vi "Dashboard Main.vi"() -> ()   [LabVIEW 2017]
uses:
  Shared/AutonomousRoutine.ctl
  <vilib>/Rock Robotics/WPI/DriverStation/WPI_DriverStationAllianceInfo.ctl
  <vilib>/Utility/miscctls.llb/LVRowAndColumnTypeDef.ctl
  <vilib>/event_ctls.llb/eventvkey.ctl
  <vilib>/Rock Robotics/WPI/Dashboard/WPI_DashboardLogging Global.vi
panel:
  in  "Camera Settings Right":T1={"Frame Rate"=30, "Compression"=30, "Size"=1, "DB Camera Config"=FALSE} {"Frame Rate" scale=1.0..30.0; "Compression" scale=100.0..-1.0; "Size" items=["640x480", "320x240", "160x120"]}
  in  "Camera Name Right":string(combo)="No Camera Selection"
  out "Camera Info":cluster{"Mbps LED":bool, "Mbps":dbl, "fps":dbl} {"fps" format="%#.1g"; "Mbps" format="%#.1g"}
  in  "Camera Settings":T1={"Frame Rate"=30, "Compression"=30, "Size"=1, "DB Camera Config"=FALSE} {"Frame Rate" scale=1.0..30.0; "Compression" scale=100.0..-1.0; "Size" items=["640x480", "320x240", "160x120"]}
  in  "TCP":refnum<k5>
  in  "Rec Mode":enum32{"Stop", "Record", "Playback"}(radio)
  out "Robot IP":string
  out "Image Message":string="Timeout in Camera Communications"
  in  "Dashboard Tab":T2(tab)
  out "NT Connection":bool
  out "Mode":T3(ring)=enum."Auto Disabled"
  out "Camera Image Right":T4(plugin-control)
  in  "DB/String 9":string
  in  "DB/String 8":string
  in  "DB/String 7":string
  in  "DB/String 6":string
  in  "DB/String 5":string
  in  "DB/String 4":string
  in  "DB/String 3":string
  in  "DB/String 2":string
  in  "DB/String 1":string
  in  "DB/String 0":string
  in  "DB/Slider 0":dbl(slide) scale=0.0..5.0
  in  "DB/Slider 1":dbl(slide) scale=0.0..5.0
  in  "DB/Slider 2":dbl(slide) scale=0.0..5.0
  in  "DB/Slider 3":dbl(slide) scale=0.0..5.0
  out "DB/LED 3":bool
  out "DB/LED 2":bool
  out "DB/LED 1":bool
  out "DB/LED 0":bool
  in  "DB/Button 3":bool
  in  "DB/Button 2":bool
  in  "DB/Button 1":bool
  in  "DB/Button 0":bool caption="New Name"
  out "Our Right Team Switch":bool
  out "Our Left Team Switch":bool
  out "Center Right Scale":bool
  out "Center Left Scale":bool
  out "Opponent Right Switch":bool
  out "Opponent Left Switch":bool
  in  "RR":T5
  in  "RL":T5
  in  "LR":T5
  in  "LL":T5
  in  "Test Slider":dbl(slide) scale=0.0..100.0 scale format="%#_3g"
  in  "On/Off":bool caption="Solenoid"
  in  "Test Name":u16(ring) items=["Select the test to run..."]
  in  "Test Tree":string(tree)
  in  "Motor":cluster{"Value":dbl, "Enable":bool} {"Value" scale=-1.0..1.0 scale format="%#_3g"}
  out "Progress":T6 {"Test Progress" scale=0.0..100.0}
  in  "Rev/Fwd":cluster{"Forward":bool, "Reverse":bool}
  in  "Test Ring":u16(ring) items=["Monochrome", "Color"]
  out "Cmd Status":string
  in  "Execute Command":bool
  in  "Command Params":string[][](table)
  in  "Command Selection":i32(listbox)
  in  "CheckList":i32(listbox)
  out "Tree":string(tree)
  out "Camera Image":T4(plugin-control)
  out "Background":bool
  in  "Camera Name":string(combo)="No Camera Selection"
  # "HW"
  # "HW"
  # "Opponent Switch"
  # "Center Scale"
  # "Our Team Switch"
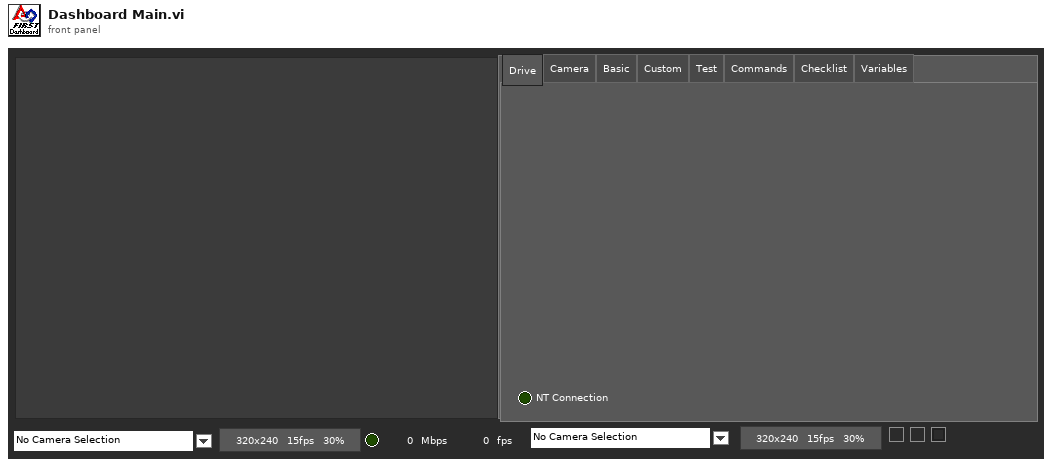
[diagram p1: front panel]
types:
  T1 = cluster{"Frame Rate":i32, "Compression":i32, "Size":u16, "DB Camera Config":bool}
  T2 = enum32{"Drive", "Camera", "Basic", "Custom", "Test", "Commands", "Checklist", "Variables"}
  T3 = enum8{"Tele-Op Disabled", "Tele-Op Enabled", "Auto Disabled", "Auto Enabled", "Test Disabled", "Test Enabled", "Disconnected", "No Code", "E-Stop"}
  T4 = typedef "IMAQ Image.ctl" = refnum<image>
  T5 = typedef "AutonomousRoutine.ctl" = enum16{"Score Scale", "Score Switch"}
  T6 = cluster{"Test Progress":u8, "Test Progress Text":string}
  T7 = cluster{"Save Path":path, "Interval (s)":dbl, "Keep":i32}
  T8 = typedef "Image Type" = u32
  T9 = cluster{"IDs":cluster{"RPC field ID":u16, "Unique ID":u16}, "String":string}
  T10 = cluster{"Error Strings":string, "Disable Counts":cluster{u16, u16}, "Rail Faults":cluster{u16, u16, u16}, "Robot IP":string, "DB Mode":u8, "Event Info":cluster{"Name":string, "Type":u8, "Number":u16, "Replay":u8}}
  T11 = cluster{"Storage":cluster{"Disk Free":u64, "RAM Block":u32, "RAM free":u32}, "CPU Utilization":cluster{"CPU % ISR":sgl, "CPU % Time Crit":sgl, "CPU % Timed Str":sgl, "CPU % High":sgl, "CPU % Above":sgl, "CPU % Normal":sgl, "CPU % Low":sgl}, "CAN":cluster{"% Bus Utilization":sgl, "Bus Off Cnt":u32, "TX_FIFO Full Cnt":u32, "Receive Error Cnt":u8, "Transmit Error Cnt":u8}, "HID":cluster{"HID Outputs":u32, "Rumble Low":u16, "Rumble High":u16}[]}
  T12 = cluster{"Status bits":cluster{"Test Mode":bool, "Autonomous":bool, "Enabled":bool, "Code Start":bool, "Brownout":bool, "Reserved 2":bool, "Reserved 3":bool, "E-Stop":bool}, "Code Trace":cluster{"Disabled":bool, "TeleOp":bool, "Auto":bool, "Test":bool}, "Controller Type":enum16{"unknown", "cRIO", "roboRio"}, "Code?":enum16{"unknown", "noCode", "code"}, "Battery V":dbl}
  T13 = cluster{"Camera Image":refnum<vi>, "Dashboard Tab":refnum<vi>, "Background":refnum<vi>, "Rec Mode":refnum<vi>, "Test Slider":refnum<vi>, "On/Off ":refnum<vi>, "Test Ring":refnum<vi>, "Rev/Fwd":refnum<vi>, "Test Name":refnum<vi>, "Motor":refnum<vi>, "Progress":refnum<vi>, "CheckList":refnum<vi>, "Tree":refnum<vi>, "Test Tree":refnum<vi>, "Command Params":refnum<vi>, "Command Selection":refnum<vi>, "Execute Command":refnum<vi>, "Cmd Status":refnum<vi>, "Camera Settings":refnum<vi>, "Camera Name":refnum<vi>, "Camera Info":refnum<vi>, "Camera Settings Right":refnum<vi>, "Camera Name Right":refnum<vi>, "Camera Image Right":refnum<vi>}
  T14 = cluster{"Camera Name":string, string, "Saved DB Images Info":cluster{"Save Path":path, "Interval (s)":dbl, "Keep":i32}}
  T15 = cluster{"Camera Name Right":string, string, "Saved DB Images Info":cluster{"Save Path":path, "Interval (s)":dbl, "Keep":i32}}
  T16 = cluster{"Operation":enum16{"Update", "Clear"}, "Color Box":u32}[]
  T17 = typedef "eventvkey.ctl" = enum16{"ASCII", "Enter", "Return", "Shift", "Ctrl", "Alt", "Cmd", "Opt", "Caps", "NumLock", "Clear", "Break", "Up", "Down", "Left", "Right", "Insert", "Delete", "Home", "End", "PageUp", "PageDown", "Escape", "Help", "Pause", "ScrollLock", "F1", "F2", "F3", "F4", "F5", "F6", "F7", "F8", "F9", "F10", "F11", "F12", "F13", "F14", "F15", "F16", "F17", "F18", "F19", "F20", "F21", "F22", "F23", "F24", "Play", "VolumeUp", "VolumeDown", "Mute", "Two Byte Char"}
  T18 = cluster{"Image Size":bool, "Image Type":bool, "Pixel Value":bool, "ROI Information":bool, "Zoom Factor":bool}
  T19 = cluster{"Operation":enum16{"Update", "Clear"}, "Color Box":u32}
  T20 = typedef "LVRowAndColumnTypeDef.ctl" = cluster{"Row":i32, "Column":i32}
  T21 = cluster{"Shift":bool, "Ctrl":bool, "Alt":bool, "Cmd":bool, "Opt":bool}
  T22 = typedef "WPI_DriverStationAllianceInfo.ctl" = enum16{"Red", "Blue", "Invalid"}
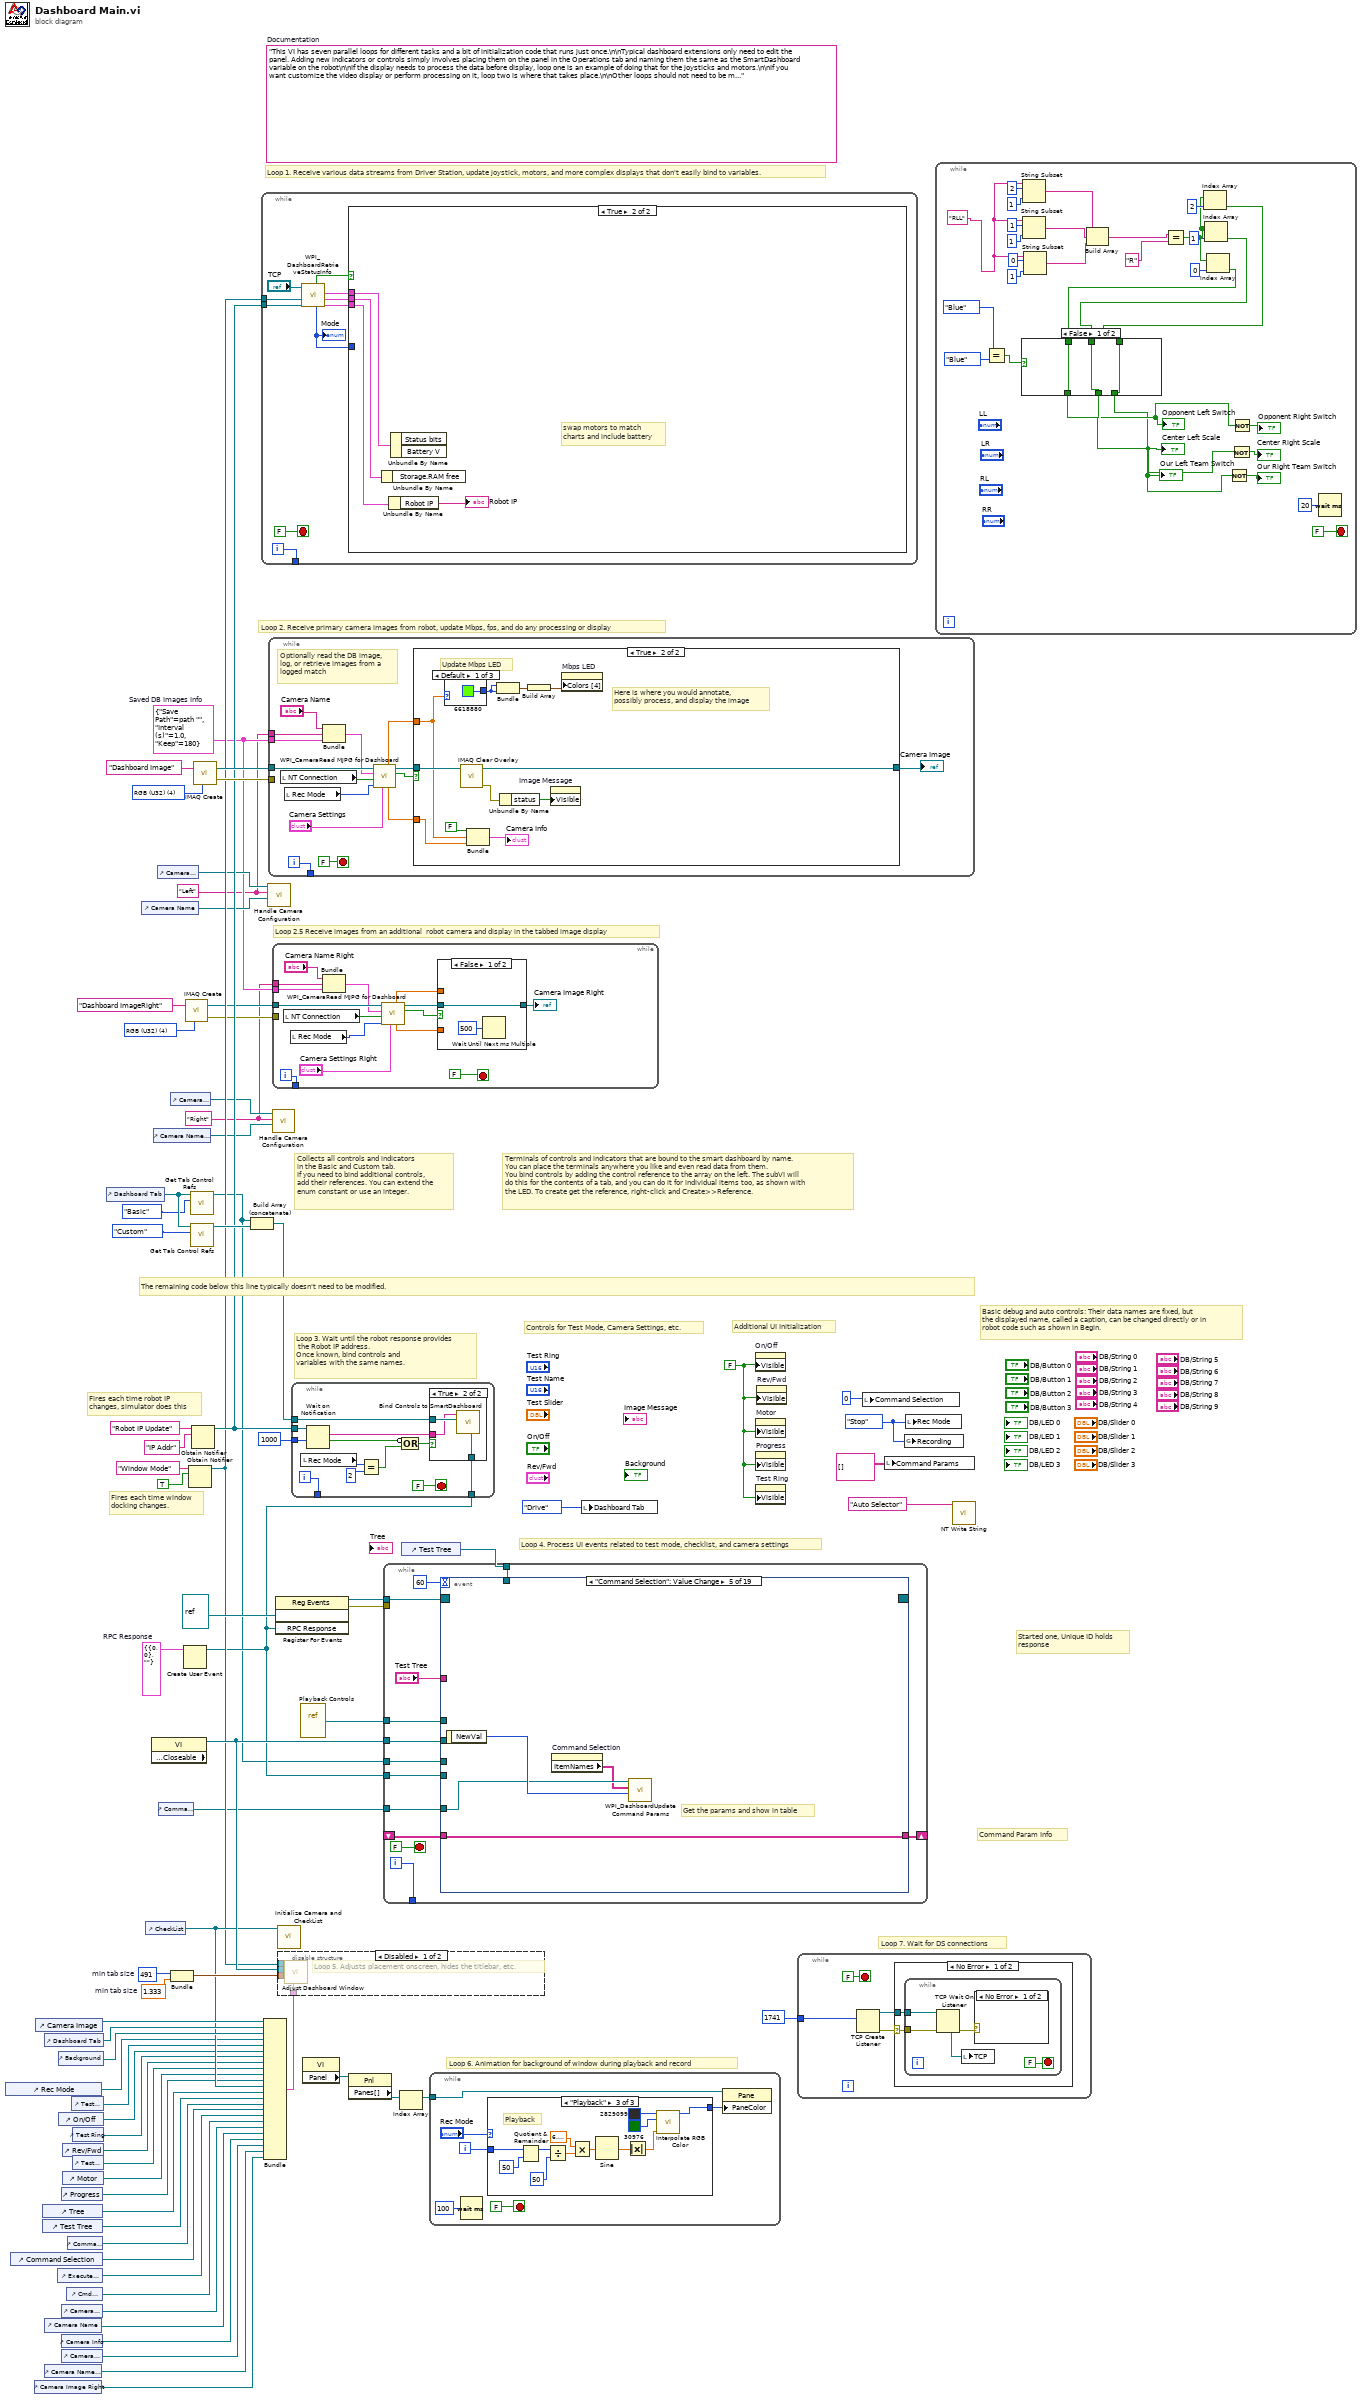
[diagram p0: block diagram]
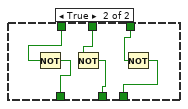
[diagram p2: hidden frame]
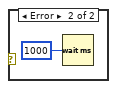
[diagram p5: hidden frame]
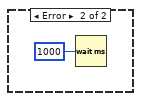
[diagram p6: hidden frame]
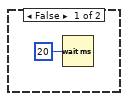
[diagram p7: hidden frame]
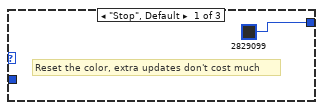
[diagram p8: hidden frame]
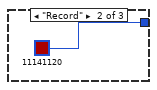
[diagram p9: hidden frame]
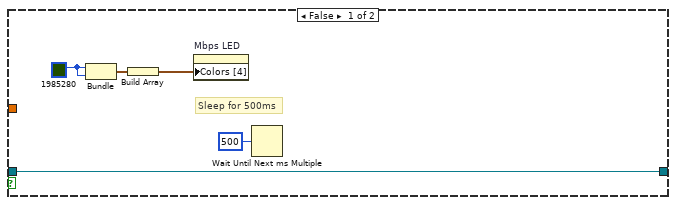
[diagram p11: hidden frame]
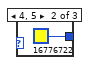
[diagram p12: hidden frame]
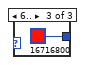
[diagram p13: hidden frame]
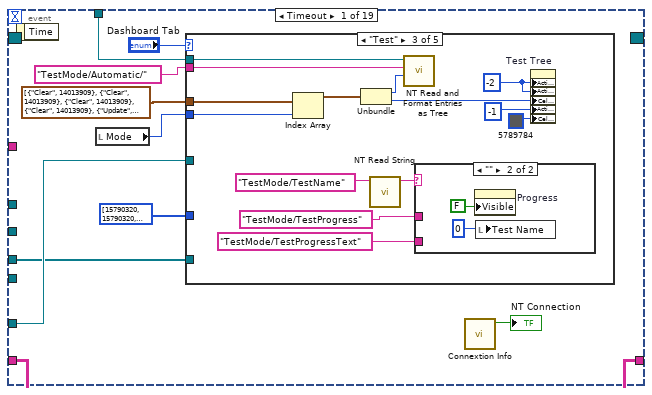
[diagram p14: hidden frame]
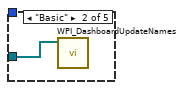
[diagram p16: hidden frame]
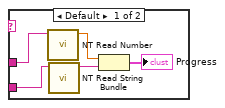
[diagram p17: hidden frame]
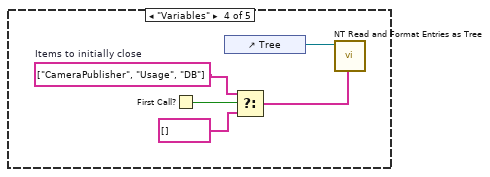
[diagram p18: hidden frame]
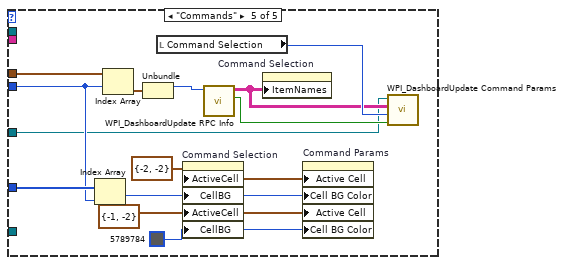
[diagram p19: hidden frame]
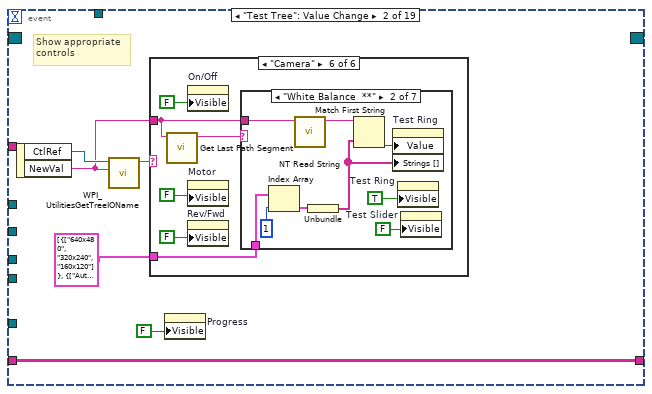
[diagram p20: hidden frame]
diagram:
  w3 = T7 {"Save Path"=path "", "Interval (s)"=1.0, "Keep"=180}  # Saved DB Images Info
  w2 = "Right"
  w1 = "Left"
  w13 = T8 4 items=["Grayscale (U8)", "Grayscale (I16)", "Grayscale (SGL)", "Complex (CSG)", "RGB (U32)", "HSL (U32)", "RGB (U64)"] ("Image Type")
  w28 = T9 {"IDs"={"RPC field ID"=0, "Unique ID"=0}, "String"=""}  # RPC Response
  w51 = 491  # min tab size
  w50 = 1.333  # min tab size
  w58 = enum32{"Stop", "Record", "Playback"}."Stop" ("Rec Mode")
  w35 = FALSE ("Visible")
  (unwired) "This VI has seven parallel loops for different tasks and a bit of initialization code that runs just once.\n\nTypical dashboard extensions only need to edit the panel. Adding new indicators or controls simply involves placing them on the panel in the Operations tab and naming them the same as the SmartDashboard variable on the robot\n\nIf the display needs to process the data before display, loop one is an example of doing that for the joysticks and motors.\n\nIf you want customize the video display or perform processing on it, loop two is where that takes place.\n\nOther loops should not need to be modified. They are pretty standard, and document the task they perform."  # Documentation
  w75 = T8 4 items=["Grayscale (U8)", "Grayscale (I16)", "Grayscale (SGL)", "Complex (CSG)", "RGB (U32)", "HSL (U32)", "RGB (U64)"] ("Image Type")
  # "Loop 2.5 Receive images from an additional  robot camera and display in the tabbed image display"
  # "Command Param Info"
  # "Started one, Unique ID holds\nresponse"
  # "Loop 7. Wait for DS connections"
  # "Basic debug and auto controls: Their data names are fixed, but\nthe displayed name, called a caption, can be changed directly or in\nrobot code such as shown in Begin."
  # "Controls for Test Mode, Camera Settings, etc."
  # "Additional UI Initialization"
  # "Loop 6. Animation for background of window during playback and record"
  # "Fires each time robot IP\nchanges, simulator does this"
  # "Fires each time window\ndocking changes."
  # "Collects all controls and indicators\nin the Basic and Custom tab.\nIf you need to bind additional controls,\nadd their references. You can extend the\nenum constant or use an integer."
  # "The remaining code below this line typically doesn't need to be modified."
  # "Loop 4. Process UI events related to test mode, checklist, and camera settings"
  # "Terminals of controls and indicators that are bound to the smart dashboard by name.\nYou can place the terminals anywhere you like and even read data from them.\nYou bind controls by adding the control reference to the array on the left. The subVI will\ndo this for the contents of a tab, and you can do it for individual items too, as shown with\nthe LED. To create get the reference, right-click and Create>>Reference."
  # "Loop 3. Wait until the robot response provides\n the Robot IP address.\nOnce known, bind controls and\nvariables with the same names."
  # "Loop 1. Receive various data streams from Driver Station, update joystick, motors, and more complex displays that don't easily bind to variables."
  # "Loop 2. Receive primary camera images from robot, update Mbps, fps, and do any processing or display"
  n1 = control-ref of="Rec Mode"() -> (w41:refnum<vi>)
  n2 = control-ref of="Command Selection"() -> (w27:refnum<vi>)
  n3 = control-ref of="Camera Image Right"() -> (w6:refnum<vi>)
  n4 = control-ref of="Camera Image"() -> (w53:refnum<vi>)
  n5 = control-ref of="Tree"() -> (w45:refnum<vi>)
  n6 = control-ref of="Test Tree"() -> (w44:refnum<vi>)
  n7 = control-ref of="Dashboard Tab"() -> (w52:refnum<vi>)
  n8 = control-ref of="Camera Name"() -> (w18:refnum<vi>)
  n9 = control-ref of="Camera Name Right"() -> (w7:refnum<vi>)
  n10 = control-ref of="Execute Command"() -> (w29:refnum<vi>)
  n11 = control-ref of="Background"() -> (w48:refnum<vi>)
  n12 = control-ref of="On/Off"() -> (w39:refnum<vi>)
  n13 = control-ref of="Progress"() -> (w36:refnum<vi>)
  n14 = control-ref of="Camera Settings"() -> (w19:refnum<vi>)
  n15 = control-ref of="Camera Info"() -> (w17:refnum<vi>)
  n16 = control-ref of="Camera Settings Right"() -> (w8:refnum<vi>)
  n17 = control-ref of="Rev/Fwd"() -> (w37:refnum<vi>)
  n18 = control-ref of="Motor"() -> (w42:refnum<vi>)
  n19 = control-ref of="Cmd Status"() -> (w23:refnum<vi>)
  n20 = control-ref of="Command Params"() -> (w30:refnum<vi>)
  n21 = control-ref of="Test Slider"() -> (w40:refnum<vi>)
  n22 = control-ref of="Test Ring"() -> (w38:refnum<vi>)
  n23 = control-ref of="Test Name"() -> (w43:refnum<vi>)
  n24 = control-ref of="Dashboard Tab"() -> (w56:refnum<vi>)
  n25 = control-ref of="Camera Name"() -> (w20:refnum<vi>)
  n26 = control-ref of="CheckList"() -> (w46:refnum<vi>)
  n27 = property class="VI" props=["Front Panel.Closeable"]() -> (reference out=w57:refnum<vi>)  [unwired: 2 in, 2 out]
  n28 = control-ref of="Camera Name Right"() -> (w9:refnum<vi>)
  n29 = control-ref of="Camera Settings"() -> (w21:refnum<vi>)
  n30 = control-ref of="Command Params"() -> (w22:refnum<vi>)
  n31 = control-ref of="Camera Settings Right"() -> (w10:refnum<vi>)
  n32 = Bundle("min tab size"=w51, "min tab size"=w50) -> (w49:cluster{"min tab size":i32, "min tab size":dbl})  [unwired: 1 in]
  n33 = Create User Event(user event datatype=w28) -> (user event=w24:refnum<user-event>)  [unwired: 1 in, 1 out]
  n34 = call "IMAQ Create"("Image Name"="Dashboard ImageRight", "Image Type"=w13) -> ("New Image"=w12:T4, "error out"=w11:errorcluster)  [unwired: 2 in, 1 out]
  n35 = Obtain Notifier(name (unnamed)="Window Mode", notification data type=TRUE) -> (notifier out=w33:refnum<notifier>)  [unwired: 2 in, 2 out]
  n36 = call <vilib>:"Get Tab Control Refs.vi"("Page Index"=T2."Basic" ("Dashboard Tab"), "TabControl in"=w56) -> ("ControlsOnPage"=w16:refnum<vi>[])  [unwired: 9 in]
  n37 = call <vilib>:"Get Tab Control Refs.vi"("Page Index"=T2."Custom" ("Dashboard Tab"), "TabControl in"=w56) -> ("ControlsOnPage"=w55:refnum<vi>[])  [unwired: 9 in]
  n38 = Obtain Notifier(name (unnamed)="Robot IP Update", notification data type="IP Addr" ("name (unnamed)")) -> (notifier out=w34:refnum<notifier>)  [unwired: 2 in, 2 out]
  n39 = call "IMAQ Create"("Image Name"="Dashboard Image", "Image Type"=w75) -> ("New Image"=w73:T4, "error out"=w72:errorcluster)  [unwired: 2 in, 1 out]
  n40 = Build Array (concatenate)(w16, w55) -> (w54:refnum<vi>[])
  n41 = while {
    tunnel: [w84] -> _
    tunnel: w34 -> [w79]
    tunnel: w33 -> [w76]
    i -> [w84]
    stop <- FALSE stop-if-true
    n42 = call <vilib>:"WPI_DashboardRetrieveStatusInfo.vi"("Binding Refnum"=w79, "Window Mode Notifier"=w76, "TCP Cnx"="TCP") -> ("Power and Errors"=w80:T10, "Robot Metrics"=w82:T11, "Status Info"=w83:T12, "Robot Mode"=w78:T3, "Process?"=w81:bool)  [unwired: 3 in, 1 out]
    "Mode" <- w78
    n43 = case shown="True" w81 {
      tunnel: w83 -> [_ w90]
      tunnel: w82 -> [_ w89]
      tunnel: w80 -> [_ w88]
      tunnel: w78 -> [_ _]
      frame False {
        n44 = Wait (ms)(milliseconds to wait=u32 20) -> ()  [unwired: 1 out]
      }
      frame True {
        # "swap motors to match\ncharts and include battery"
        n45 = Unbundle By Name(w89) -> ()  [unwired: 1 out]
        n46 = Unbundle By Name(w88) -> ("Robot IP"=→"Robot IP":string)
        n47 = Unbundle By Name(w90) -> ()  [unwired: 2 out]
      }
    }
  }
  n48 = Bundle("Camera Image"=w53, "Dashboard Tab"=w52, "Background"=w48, "Rec Mode"=w41, "Test Slider"=w40, "On/Off"=w39, "Test Ring"=w38, "Rev/Fwd"=w37, "Test Name"=w43, "Motor"=w42, "Progress"=w36, "CheckList"=w46, "Tree"=w45, "Test Tree"=w44, "Command Params"=w30, "Command Selection"=w27, "Execute Command"=w29, "Cmd Status"=w23, "Camera Settings"=w19, "Camera Name"=w18, "Camera Info"=w17, "Camera Settings Right"=w8, "Camera Name Right"=w7, "Camera Image Right"=w6) -> (w47:T13)  [unwired: 1 in]
  n49 = call "Handle Camera Configuration.vi"("CameraNameRef"=w20, "Display Name"=w1, "ClusterRef"=w21) -> ()  [unwired: 9 in]
  n50 = while {
    tunnel: w73 -> [w103]
    tunnel: w72 -> [_]
    tunnel: [w104] -> _
    tunnel: w3 -> [w94]
    tunnel: w1 -> [w91]
    i -> [w104]
    stop <- FALSE stop-if-true
    # "Optionally read the DB image,\nlog, or retrieve images from a\nlogged match"
    n51 = local read "NT Connection"() -> (w95:bool)
    n52 = local read "Rec Mode"() -> (w99:enum32{"Stop", "Record", "Playback"})
    n53 = Bundle("Camera Name"="Camera Name", w91, "Saved DB Images Info"=w94) -> (w93:T14)  [unwired: 1 in]
    n54 = call <vilib>:"WPI_CameraRead MJPG for Dashboard.vi"("Camera Settings"="Camera Settings", "Rec Mode"=w99, "NT Connection"=w95, "Capture Info"=w93, "Refnum in"=w103) -> ("Active"=w101:bool, "Refnum out"=w102:T4, "FPS"=w100:dbl, "Bandwidth (Mbps)"=w98:dbl)  [unwired: 3 in]
    n55 = case shown="True" w101 {
      tunnel: w102 -> [w106 w117]
      tunnel: w98 -> [_ w114]
      tunnel: w100 -> [_ w115]
      tunnel: [w106 w111] -> w96
      frame False {
        w108 = u32 1985280 ("Color Box")
        # "Sleep for 500ms"
        n56 = Bundle("Color Box"=w108, "Color Box"=w108) -> (w109:cluster{"Color Box":u32, "Color Box":u32})  [unwired: 1 out]
        n57 = Build Array(w109) -> (w107:cluster{"Color Box":u32, "Color Box":u32}[])
        n58 = property on="Mbps LED" class="Bool (strict)"("Colors [4]"=w107) -> ()  [unwired: 2 in, 2 out]
        n59 = Wait Until Next ms Multiple(millisecond multiple=u32 500) -> ()  [unwired: 1 out]
      }
      frame True {
        # "Here is where you would annotate,\npossibly process, and display the image"
        # "Update Mbps LED"
        n60 = case shown="Default" w114 {
          tunnel: [u32 6618880 ("Color Box") u32 16776722 ("Color Box") u32 16716800 ("Color Box")] -> w118
          frame Default {
          }
          frame 4, 5 {
          }
          frame 6.. {
          }
        }
        n61 = call "IMAQ Clear Overlay"("Image"=w117) -> ("error out"=w120:errorcluster, "Image Out"=w111:T4)  [unwired: 2 in, 7 out]
        n62 = Bundle(FALSE, "Bandwidth (Mbps)"=w114, "FPS"=w115) -> (→"Camera Info":cluster{bool, "Bandwidth (Mbps)":dbl, "FPS":dbl})  [unwired: 1 in]
        n63 = Bundle("Color Box"=w118, "Color Box"=w118) -> (w119:cluster{"Color Box":u32, "Color Box":u32})  [unwired: 1 out]
        n64 = Unbundle By Name(w120) -> ("status"=w121:bool)
        n65 = Build Array(w119) -> (w116:cluster{"Color Box":u32, "Color Box":u32}[])
        n66 = property on="Image Message" class="Str"("Visible"=w121) -> ()  [unwired: 2 in, 2 out]
        n67 = property on="Mbps LED" class="Bool (strict)"("Colors [4]"=w116) -> ()  [unwired: 2 in, 2 out]
      }
    }
    "Camera Image" <- w96
  }
  n68 = call "Handle Camera Configuration.vi"("CameraNameRef"=w9, "Display Name"=w2, "ClusterRef"=w10) -> ()  [unwired: 9 in]
  n69 = while {
    tunnel: w12 -> [w139]
    tunnel: w11 -> [_]
    tunnel: [w134] -> _
    tunnel: w3 -> [w128]
    tunnel: w2 -> [w125]
    i -> [w134]
    stop <- FALSE stop-if-true
    n70 = local read "NT Connection"() -> (w129:bool)
    n71 = local read "Rec Mode"() -> (w138:enum32{"Stop", "Record", "Playback"})
    n72 = Bundle("Camera Name Right"="Camera Name Right", w125, "Saved DB Images Info"=w128) -> (w127:T15)  [unwired: 1 in]
    n73 = call <vilib>:"WPI_CameraRead MJPG for Dashboard.vi"("Camera Settings"="Camera Settings Right", "Rec Mode"=w138, "NT Connection"=w129, "Capture Info"=w127, "Refnum in"=w139) -> ("Active"=w133:bool, "Refnum out"=w136:T4, "FPS"=w131:dbl, "Bandwidth (Mbps)"=w132:dbl)  [unwired: 3 in]
    n74 = case shown="False" w133 {
      tunnel: w136 -> [w140 w142]
      tunnel: w132 -> [_ _]
      tunnel: w131 -> [_ _]
      tunnel: [w140 w142] -> w130
      frame False {
        n75 = Wait Until Next ms Multiple(millisecond multiple=u32 500) -> ()  [unwired: 1 out]
      }
      frame True {
      }
    }
    "Camera Image Right" <- w130
  }
  n76 = register-events(refnum<vi> refnum, w24) -> (reference out=w62:refnum<event-registration>, error out=w61:errorcluster)  [unwired: 2 in]
  n77 = call "Initialize Camera and CheckList.vi"("ListBox in"=w46) -> ()  [unwired: 11 in]
  n78 = disable-structure shown="Disabled" {
    disable-tunnel: w57 -> [w146 _]
    disable-tunnel: w49 -> [w145 _]
    disable-tunnel: w47 -> [w144 _]
    disable-tunnel: w33 -> [w143 _]
    frame Disabled {
      # "Loop 5. Adjusts placement onscreen, hides the titlebar, etc."
      n79 = call "Adjust Dashboard Window.vi"("Sizing Refnums"=w144, "Size Constraints"=w145, "VI"=w146, "WIn Mode"=w143) -> ()  [unwired: 8 in]
    }
    frame Enabled {
    }
  }
  n80 = while {
    tunnel: w54 -> [w158]
    tunnel: w34 -> [w156]
    tunnel: [w154] -> _
    tunnel: u32 1000 ("milliseconds to wait") -> [w153]
    tunnel: w24 -> [w147]
    i -> [w154]
    stop <- FALSE stop-if-true
    n81 = local read "Rec Mode"() -> (w149:enum32{"Stop", "Record", "Playback"})
    n82 = Wait on Notification(notifier=w156, timeout in ms (-1)=w153) -> (notification=w155:string, timed out?=w151:bool)  [unwired: 2 in, 2 out]
    n83 = Equal?(x=w149, y=u16 2 ("Rec Mode")) -> (x = y?=w150:bool)
    n84 = Compound Arithmetic op=OR(invert w151, w150) -> (w152:bool)
    n85 = case shown="True" w152 {
      tunnel: w158 -> [_ w161]
      tunnel: w155 -> [_ w160]
      tunnel: w147 -> [_ w159]
      frame False {
      }
      frame True {
        n86 = call <vilib>:"Bind Controls to SmartDashboard.vi"("RPC ref"=w159, "Bound Control Refs"=w161, "Server IP Address"=w160) -> ()  [unwired: 9 in]
      }
    }
  }
  n87 = vi-ref "Playback Controls.vi"() -> (w63:refnum<vi>)
  n88 = property class="VI"() -> ("Panel"=w65:refnum<vi>)  [unwired: 2 in, 2 out]
  n89 = property class="Pnl"(reference=w65) -> ("Panes[]"=w66:refnum<vi>[])  [unwired: 1 in, 2 out]
  n90 = Index Array(array=w66) -> (element=w64:refnum<vi>)  [unwired: 1 in]
  n91 = control-ref of="Test Tree"() -> (w67:refnum<vi>)
  n92 = while {
    tunnel: [w171] -> _
    tunnel: w67 -> [w170]
    tunnel: w63 -> [w169]
    tunnel: w62 -> [w168]
    tunnel: w61 -> [_]
    tunnel: w57 -> [w167]
    tunnel: w24 -> [w166]
    tunnel: w22 -> [w165]
    shift-right: [w164] -> _
    shift-left: _ -> [w163]
    tunnel: w16 -> [w162]
    i -> [w171]
    stop <- FALSE stop-if-true
    n93 = event shown="[4] \"Command Selection\": Value Change" {
      selector: w168 -> [_ _ _ _ _ _ _ _ _ _ _ _ _ _ _ _ _ _ _]
      dyn-events: [_ _ _ _ _ _ _ _ _ _ _ _ _ _ w425 _ _ _ _] -> _
      timeout: u32 60 ("milliseconds to wait") -> [_ _ _ _ _ _ _ _ _ _ _ _ _ _ _ _ _ _ _]
      tunnel: w170 -> [w183 _ _ _ _ _ _ _ _ _ _ _ _ _ _ _ _ _ _]
      tunnel: "Test Tree" -> [_ _ _ _ _ _ _ _ _ w392 w400 w402 w406 w414 _ _ _ _ _]
      tunnel: w169 -> [_ _ _ _ _ _ _ _ _ _ _ _ _ _ w427 _ w445 _ _]
      tunnel: w167 -> [_ _ _ _ _ _ _ _ _ _ _ _ _ _ w423 _ _ _ _]
      tunnel: w166 -> [_ _ _ _ _ _ _ _ _ _ _ _ _ _ w421 _ _ _ _]
      tunnel: w165 -> [w178 _ _ _ w343 _ _ _ _ _ _ _ _ _ _ _ _ _ _]
      tunnel: [w177 w226 w328 w333 w341 w350 w360 w367 w379 w391 w398 w401 w405 w413 w420 w440 w442 w446 w459] -> w164
      tunnel: w163 -> [w177 w226 w328 w333 w341 _ _ w367 w379 w391 w398 w401 w405 w413 w420 w440 w442 w446 w459]
      tunnel: w162 -> [w175 _ _ _ _ _ _ _ _ _ _ _ _ _ _ _ _ _ _]
      event Timeout {
        n94 = event-data() -> ()  [unwired: 1 in, 1 out]
        n95 = local read "Mode"() -> (w180:T3)
        n96 = case shown="\"Test\"" "Dashboard Tab" {
          tunnel: w183 -> [_ _ w199 _ _]
          tunnel: "TestMode/Automatic/" ("Name Pattern") -> [_ _ w198 _ _]
          tunnel: T16 [{"Operation"=enum."Clear", "Color Box"=14013909}, {"Operation"=enum."Clear", "Color Box"=14013909}, {"Operation"=enum."Clear", "Color Box"=14013909}, {"Operation"=enum."Clear", "Color Box"=14013909}, {"Operation"=enum."Update", "Color Box"=14013909}, {"Operation"=enum."Update", "Color Box"=16777215}, {"Operation"=enum."Clear", "Color Box"=14013909}, {"Operation"=enum."Clear", "Color Box"=14013909}, {"Operation"=enum."Clear", "Color Box"=14013909}] -> [_ _ w191 _ w219]
          tunnel: w180 -> [_ _ w190 _ w218]
          tunnel: u32[] [15790320, 15790320, 15790320, 15790320, 16777215, 16777215, 15790320, 15790320, 15790320] -> [_ _ _ _ w224]
          tunnel: w178 -> [_ _ _ _ w212]
          tunnel: w175 -> [_ w185 _ _ _]
          frame "Custom", Default {
          }
          frame "Basic" {
            n97 = call <vilib>:"WPI_DashboardUpdateNames.vi"("Controls on Tab"=w185) -> ()  [unwired: 11 in]
          }
          frame "Test" {
            w197 = -2 ("Active Item:Row Number")
            n98 = Index Array(array=w191, index=w190) -> (element=w192:T19)
            n99 = Unbundle(w192) -> ("Operation"=w193:enum16{"Update", "Clear"}, "Color Box"=w194:u32)
            n100 = call <vilib>:"NT Read String.vi"("Name"="TestMode/TestName") -> ("String"=w188:string)  [unwired: 9 in, 1 out]
            n101 = call <vilib>:"NT Read and Format Entries as Tree.vi"("Operation"=w193, "Name Pattern"=w198, "Tree Refnum"=w199) -> ()  [unwired: 7 in, 2 out]
            n102 = case shown="\"\"" w188 {
              tunnel: "TestMode/TestProgress" ("Name") -> [w201 _]
              tunnel: "TestMode/TestProgressText" ("Name") -> [w200 _]
              frame Default {
                n103 = call <vilib>:"NT Read Number.vi"("Name"=w201) -> ("Numeric"=w202:dbl)  [unwired: 9 in, 1 out]
                n104 = call <vilib>:"NT Read String.vi"("Name"=w200) -> ("String"=w203:string)  [unwired: 9 in, 1 out]
                n105 = Bundle("Numeric"=w202, "String"=w203) -> (→"Progress":cluster{"Numeric":dbl, "String":string})  [unwired: 1 in]
              }
              frame "" {
                n106 = property on="Progress" class="Clust (strict)"("Visible"=FALSE) -> ()  [unwired: 2 in, 2 out]
                n107 = local write "Test Name"(u16 0) -> ()
              }
            }
            n108 = property on="Test Tree" class="Tree (strict)"("Active Item Row Number"=w197, "ActiveColNum"=w197, "CellBG"=w194, "Active Item Row Number"=-1 ("Active Item:Row Number"), "CellBG"=u32 5789784 ("Color Box")) -> ()  [unwired: 2 in, 2 out]
          }
          frame "Variables" {
            w209 = string[] ["CameraPublisher", "Usage", "DB"]  # Items to initially close
            n109 = First Call?() -> (First Call?: T/F=w210:bool)
            n110 = control-ref of="Tree"() -> (w211:refnum<vi>)
            n111 = Select(t=w209, s=w210, f=string[] []) -> (s? t:f=w207:string[])
            n112 = call <vilib>:"NT Read and Format Entries as Tree.vi"("Tags to  Close"=w207, "Tree Refnum"=w211) -> ()  [unwired: 8 in, 2 out]
          }
          frame "Commands" {
            w220 = u32 5789784 ("Color Box")
            w221 = T20 {"Row"=-1, "Column"=-2} ("Active Cell:Active Cell")
            w223 = T20 {"Row"=-2, "Column"=-2} ("Active Cell:Active Cell")
            n113 = Index Array(array=w224, index=w218) -> (element=w222:u32)
            n114 = Index Array(array=w219, index=w218) -> (element=w217:T19)
            n115 = Unbundle(w217) -> ("Operation"=w216:enum16{"Update", "Clear"})  [unwired: 1 out]
            n116 = local read "Command Selection"() -> (w215:i32)
            n117 = property on="Command Selection" class="MCListbox (strict)"("ActiveCell"=w223, "CellBG"=w222, "ActiveCell"=w221, "CellBG"=w220) -> ()  [unwired: 2 in, 2 out]
            n118 = call <vilib>:"WPI_DashboardUpdate RPC Info.vi"("Operation"=w216) -> ("update"=w214:bool, "commands"=w213:string[][])  [unwired: 9 in]
            n119 = property on="Command Selection" class="MCListbox (strict)"("ItemNames"=w213) -> ()  [unwired: 2 in, 2 out]
            n120 = property on="Command Params" class="Tbl (strict)"("Active Cell"=w223, "Cell BG Color"=w222, "Active Cell"=w221, "Cell BG Color"=w220) -> ()  [unwired: 2 in, 2 out]
            n121 = call <vilib>:"WPI_DashboardUpdate Command Params.vi"("Update"=w214, "NewVal"=w215, "Commands"=w213, "Param Tbl"=w212) -> ()  [unwired: 7 in, 1 out]
          }
        }
        n122 = call <vilib>:"Connextion Info.vi"() -> ("Connected"=→"NT Connection":bool)  [unwired: 10 in, 1 out]
      }
      event "Test Tree": Value Change {
        # "Show appropriate\ncontrols"
        n123 = event-data() -> ("CtlRef"=w229:refnum<vi>, "NewVal"=w227:string)  [unwired: 1 in]
        n124 = call <vilib>:"WPI_UtilitiesGetTreeIOName.vi"("NewVal"=w227, "TreeControl in"=w229) -> ("I/O Name"=w230:string)  [unwired: 9 in]
        n125 = case shown="\"Camera\"" w230 {
          selector: w230 -> [_ w237 _ w259 w268 _]
          tunnel: w227 -> [_ _ w256 w258 _ w275]
          tunnel: cluster{string[]}[] [{["640x480", "320x240", "160x120"]}, {["Auto", "Fixed indoor", "Fixed outdoor 1", "Fixed outdoor 2", "Fixed fluorescent 1", "Fixed fluorescent 2", "Hold current"]}, {["Auto", "Flicker-free 50 Hz", "Flicker-free 60 Hz", "Hold current"]}, {["None", "Prioritize frame rate", "Prioritize image quality"]}, {["Monochrome", "Color"]}] -> [_ _ _ _ _ w274]
          frame Default {
            w232 = FALSE ("Visible")
            w231 = FALSE ("Visible")
            n126 = property on="Motor" class="Clust (strict)"("Visible"=w231) -> ()  [unwired: 2 in, 2 out]
            n127 = property on="Test Ring" class="Ring (strict)"("Visible"=w231) -> ()  [unwired: 2 in, 2 out]
            n128 = property on="Rev/Fwd" class="Clust (strict)"("Visible"=w232) -> ()  [unwired: 2 in, 2 out]
            n129 = property on="On/Off" class="Bool (strict)"("Visible"=w232) -> ()  [unwired: 2 in, 2 out]
            n130 = property on="Test Slider" class="Slide (strict)"("Visible"=w232) -> ()  [unwired: 2 in, 2 out]
          }
          frame "Analog Out", "Motor", "PWM" {
            w238 = FALSE ("Visible")
            n131 = case shown="\"Analog Out\"" w237 {
              tunnel: [1.0 ("Value") -1.0 ("Value") 0.0 ("Value")] -> w236
              tunnel: [255.0 ("Value") 1.0 ("Value") 5.0 ("Value")] -> w235
              tunnel: [128.0 ("Value") 0.0 ("Value") 0.0 ("Value")] -> w234
              tunnel: [64.0 ("Value") 0.5 ("Value") 1.0 ("Value")] -> w233
              frame "PWM" {
              }
              frame "Motor", Default {
              }
              frame "Analog Out" {
              }
            }
            n132 = property on="Motor" class="Clust (strict)"("Visible"=TRUE) -> ()  [unwired: 2 in, 2 out]
            n133 = property on="Value" class="Slide (strict)"("Value"=w234, "Scale.Minimum"=w236, "Scale.Maximum"=w235, "Scale.Increment"=w233) -> ()  [unwired: 2 in, 2 out]
            n134 = property on="On/Off" class="Bool (strict)"("Visible"=w238) -> ()  [unwired: 2 in, 2 out]
            n135 = property on="Test Slider" class="Slide (strict)"("Visible"=w238) -> ()  [unwired: 2 in, 2 out]
            n136 = property on="Test Ring" class="Ring (strict)"("Visible"=w238) -> ()  [unwired: 2 in, 2 out]
            n137 = property on="Rev/Fwd" class="Clust (strict)"("Visible"=w238) -> ()  [unwired: 2 in, 2 out]
          }
          frame "Servo" {
            w254 = FALSE ("Visible")
            n138 = call <vilib>:"NT Read Number.vi"("Name"=w256) -> ("Numeric"=w255:dbl)  [unwired: 9 in, 1 out]
            n139 = property on="Test Slider" class="Slide (strict)"("Visible"=TRUE, "Scale.Maximum"=170.0 ("Scale.Range:Maximum")) -> ()  [unwired: 2 in, 2 out]
            n140 = local write "Test Slider"(w255) -> ()
            n141 = property on="Motor" class="Clust (strict)"("Visible"=w254) -> ()  [unwired: 2 in, 2 out]
            n142 = property on="Rev/Fwd" class="Clust (strict)"("Visible"=w254) -> ()  [unwired: 2 in, 2 out]
            n143 = property on="On/Off" class="Bool (strict)"("Visible"=w254) -> ()  [unwired: 2 in, 2 out]
            n144 = property on="Test Ring" class="Ring (strict)"("Visible"=w254) -> ()  [unwired: 2 in, 2 out]
          }
          frame "Relay", "Solenoid" {
            w257 = FALSE ("Visible")
            n145 = property on="Motor" class="Clust (strict)"("Visible"=w257) -> ()  [unwired: 2 in, 2 out]
            n146 = property on="Test Slider" class="Slide (strict)"("Visible"=w257) -> ()  [unwired: 2 in, 2 out]
            n147 = Search and Replace String(input string=w258, search string="/Value  **", replace string="/Direction") -> (result string=w264:string)  [unwired: 5 in, 3 out]
            n148 = property on="Test Ring" class="Ring (strict)"("Visible"=w257) -> ()  [unwired: 2 in, 2 out]
            n149 = call <vilib>:"NT Read String.vi"("Name"=w264) -> ("String"=w262:string)  [unwired: 9 in, 1 out]
            n150 = Equal?(x="Both directions", y=w262) -> (x = y?=w260:bool)
            n151 = Not(x=w260) -> (.not. x?=w261:bool)
            n152 = property on="Rev/Fwd" class="Clust (strict)"("Visible"=w260) -> ()  [unwired: 2 in, 2 out]
            n153 = property on="On/Off" class="Bool (strict)"("Visible"=w261, "Caption.Text"=w259) -> ()  [unwired: 2 in, 2 out]
          }
          frame "Compressor", "Digital Out" {
            w267 = FALSE ("Visible")
            # "Get direction and finish"
            n154 = property on="Motor" class="Clust (strict)"("Visible"=w267) -> ()  [unwired: 2 in, 2 out]
            n155 = property on="Test Slider" class="Slide (strict)"("Visible"=w267) -> ()  [unwired: 2 in, 2 out]
            n156 = property on="Test Ring" class="Ring (strict)"("Visible"=w267) -> ()  [unwired: 2 in, 2 out]
            n157 = property on="On/Off" class="Bool (strict)"("Visible"=TRUE, "Caption.Text"=w268) -> ()  [unwired: 2 in, 2 out]
            n158 = property on="Rev/Fwd" class="Clust (strict)"("Visible"=FALSE) -> ()  [unwired: 2 in, 2 out]
          }
          frame "Camera" {
            n159 = call <vilib>:"Get Last Path Segment.vi"("String in"=w275) -> ("String out"=w276:string)  [unwired: 10 in]
            n160 = property on="On/Off" class="Bool (strict)"("Visible"=FALSE) -> ()  [unwired: 2 in, 2 out]
            n161 = property on="Motor" class="Clust (strict)"("Visible"=FALSE) -> ()  [unwired: 2 in, 2 out]
            n162 = property on="Rev/Fwd" class="Clust (strict)"("Visible"=FALSE) -> ()  [unwired: 2 in, 2 out]
            n163 = case shown="\"White Balance  **\"" w276 {
              tunnel: w275 -> [w282 w291 w300 w309 w318 _ w324]
              tunnel: w274 -> [w280 w288 w297 w306 w315 _ _]
              frame "Size  **" {
                n164 = Index Array(array=w280) -> (element=w279:cluster{string[]})  [unwired: 1 in]
                n165 = call <vilib>:"NT Read String.vi"("Name"=w282) -> ("String"=w281:string)  [unwired: 9 in, 1 out]
                n166 = Unbundle(w279) -> (w277:string[])
                n167 = Match First String(2:w277, 3:w281) -> (0:w278:i32)  [unwired: 1 out]
                n168 = property on="Test Ring" class="Ring (strict)"("Value"=w278, "Strings []"=w277) -> ()  [unwired: 2 in, 2 out]
                n169 = property on="Test Ring" class="Ring (strict)"("Visible"=TRUE) -> ()  [unwired: 2 in, 2 out]
                n170 = property on="Test Slider" class="Slide (strict)"("Visible"=FALSE) -> ()  [unwired: 2 in, 2 out]
              }
              frame "White Balance  **" {
                n171 = Index Array(array=w288, index=1) -> (element=w289:cluster{string[]})
                n172 = call <vilib>:"NT Read String.vi"("Name"=w291) -> ("String"=w290:string)  [unwired: 9 in, 1 out]
                n173 = Unbundle(w289) -> (w286:string[])
                n174 = Match First String(2:w286, 3:w290) -> (0:w285:i32)  [unwired: 1 out]
                n175 = property on="Test Ring" class="Ring (strict)"("Value"=w285, "Strings []"=w286) -> ()  [unwired: 2 in, 2 out]
                n176 = property on="Test Ring" class="Ring (strict)"("Visible"=TRUE) -> ()  [unwired: 2 in, 2 out]
                n177 = property on="Test Slider" class="Slide (strict)"("Visible"=FALSE) -> ()  [unwired: 2 in, 2 out]
              }
              frame "Exposure  **" {
                n178 = Index Array(array=w297, index=2) -> (element=w298:cluster{string[]})
                n179 = call <vilib>:"NT Read String.vi"("Name"=w300) -> ("String"=w299:string)  [unwired: 9 in, 1 out]
                n180 = Unbundle(w298) -> (w294:string[])
                n181 = Match First String(2:w294, 3:w299) -> (0:w295:i32)  [unwired: 1 out]
                n182 = property on="Test Ring" class="Ring (strict)"("Value"=w295, "Strings []"=w294) -> ()  [unwired: 2 in, 2 out]
                n183 = property on="Test Ring" class="Ring (strict)"("Visible"=TRUE) -> ()  [unwired: 2 in, 2 out]
                n184 = property on="Test Slider" class="Slide (strict)"("Visible"=FALSE) -> ()  [unwired: 2 in, 2 out]
              }
              frame "Exposure Priority  **" {
                n185 = Index Array(array=w306, index=3) -> (element=w307:cluster{string[]})
                n186 = call <vilib>:"NT Read String.vi"("Name"=w309) -> ("String"=w308:string)  [unwired: 9 in, 1 out]
                n187 = Unbundle(w307) -> (w303:string[])
                n188 = Match First String(2:w303, 3:w308) -> (0:w304:i32)  [unwired: 1 out]
                n189 = property on="Test Ring" class="Ring (strict)"("Value"=w304, "Strings []"=w303) -> ()  [unwired: 2 in, 2 out]
                n190 = property on="Test Ring" class="Ring (strict)"("Visible"=TRUE) -> ()  [unwired: 2 in, 2 out]
                n191 = property on="Test Slider" class="Slide (strict)"("Visible"=FALSE) -> ()  [unwired: 2 in, 2 out]
              }
              frame "Color Enable  **" {
                n192 = Index Array(array=w315, index=4) -> (element=w316:cluster{string[]})
                n193 = call <vilib>:"NT Read String.vi"("Name"=w318) -> ("String"=w317:string)  [unwired: 9 in, 1 out]
                n194 = Unbundle(w316) -> (w312:string[])
                n195 = Match First String(2:w312, 3:w317) -> (0:w313:i32)  [unwired: 1 out]
                n196 = property on="Test Ring" class="Ring (strict)"("Value"=w313, "Strings []"=w312) -> ()  [unwired: 2 in, 2 out]
                n197 = property on="Test Ring" class="Ring (strict)"("Visible"=TRUE) -> ()  [unwired: 2 in, 2 out]
                n198 = property on="Test Slider" class="Slide (strict)"("Visible"=FALSE) -> ()  [unwired: 2 in, 2 out]
              }
              frame Default {
                n199 = property on="Test Ring" class="Ring (strict)"("Visible"=FALSE) -> ()  [unwired: 2 in, 2 out]
                n200 = property on="Test Slider" class="Slide (strict)"("Visible"=FALSE) -> ()  [unwired: 2 in, 2 out]
              }
              frame "Brightness  **", "Color Level  **", "Compression  **", "FPS  **", "Sharpness  **" {
                n201 = call <vilib>:"NT Read Number.vi"("Name"=w324) -> ("Numeric"=w323:dbl)  [unwired: 9 in, 1 out]
                n202 = local write "Test Slider"(w323) -> ()
                n203 = property on="Test Slider" class="Slide (strict)"("Visible"=TRUE, "Scale.Maximum"=100.0 ("Scale.Range:Maximum")) -> ()  [unwired: 2 in, 2 out]
                n204 = property on="Test Ring" class="Ring (strict)"("Visible"=FALSE) -> ()  [unwired: 2 in, 2 out]
              }
            }
          }
        }
        n205 = property on="Progress" class="Clust (strict)"("Visible"=FALSE) -> ()  [unwired: 2 in, 2 out]
      }
      event "Test Name": Mouse Enter {
        # "Populate the ring with the list of tests"
        n206 = event-data() -> ()  [unwired: 1 in, 1 out]
        n207 = call <vilib>:"NT Read String Array.vi"("Name"="TestMode/TestList") -> ("String Array"=w332:string[])  [unwired: 9 in, 1 out]
        n208 = Build Array (concatenate)("Select the test to run...", w332) -> (w331:string[])
        n209 = property on="Test Name" class="Ring (strict)"("Strings []"=w331) -> ()  [unwired: 2 in, 2 out]
      }
      event "Test Name": Value Change {
        w334 = FALSE ("Visible")
        # "Tell the robot the test name to run"
        n210 = event-data() -> ("NewVal"=w338:u16)  [unwired: 1 in]
        n211 = property on="Test Name" class="Ring (strict)"() -> ("Strings []"=w339:string[])  [unwired: 2 in, 2 out]
        n212 = local write "Progress"(T6 {"Test Progress"=0, "Test Progress Text"=""} ("Progress")) -> ()
        n213 = Index Array(array=w339, index=w338) -> (element=w337:string)
        n214 = call <vilib>:"NT Write String.vi"("String"=w337, "Name"="TestMode/TestName") -> ()  [unwired: 9 in, 1 out]
        n215 = property on="Progress" class="Clust (strict)"("Visible"=TRUE) -> ()  [unwired: 2 in, 2 out]
        n216 = property on="Motor" class="Clust (strict)"("Visible"=w334) -> ()  [unwired: 2 in, 2 out]
        n217 = property on="Test Slider" class="Slide (strict)"("Visible"=w334) -> ()  [unwired: 2 in, 2 out]
        n218 = property on="On/Off" class="Bool (strict)"("Visible"=w334) -> ()  [unwired: 2 in, 2 out]
        n219 = property on="Rev/Fwd" class="Clust (strict)"("Visible"=w334) -> ()  [unwired: 2 in, 2 out]
        n220 = property on="Test Ring" class="Ring (strict)"("Visible"=w334) -> ()  [unwired: 2 in, 2 out]
      }
      event "Command Selection": Value Change {
        # "Get the params and show in table"
        n221 = event-data() -> ("NewVal"=w344:i32)  [unwired: 1 in]
        n222 = property on="Command Selection" class="MCListbox (strict)"() -> ("ItemNames"=w342:string[][])  [unwired: 2 in, 2 out]
        n223 = call <vilib>:"WPI_DashboardUpdate Command Params.vi"("NewVal"=w344, "Commands"=w342, "Param Tbl"=w343) -> ()  [unwired: 8 in, 1 out]
      }
      event "Execute Command": Value Change {
        # "Started one, Unique ID holds\nresponse"
        n224 = event-data() -> ()  [unwired: 1 in, 1 out]
        n225 = property on="Command Selection" class="MCListbox (strict)"() -> ("ItemNames"=w355:string[][])  [unwired: 2 in, 2 out]
        n226 = Index Array(array=w355, index (row)="Command Selection", index (col)=0) -> (element=w353:string)
        n227 = call <vilib>:"Invoke Commands.vi"("Command Params"="Command Params", "Function Name"=w353) -> ("Params"=w349:u8, "Started"=w348:bool)  [unwired: 7 in, 1 out]
        n228 = Array Subset(array="Command Params", length (row)=w349) -> (w350:string[][])  [unwired: 3 in]
        n229 = Select(t="Executing" ("Cmd Status"), s=w348, f="" ("Cmd Status")) -> (s? t:f=→"Cmd Status":string)
      }
      event "Command Selection": Double Click {
        n230 = event-data() -> ("Row"=w363:i32)  [unwired: 1 in]
        n231 = property on="Command Selection" class="MCListbox (strict)"() -> ("ItemNames"=w366:string[][])  [unwired: 2 in, 2 out]
        n232 = local read "Command Params"() -> (w362:string[][])
        n233 = Index Array(array=w366, index (row)=w363, index (col)=0) -> (element=w364:string)
        n234 = call <vilib>:"Invoke Commands.vi"("Command Params"=w362, "Function Name"=w364) -> ("Params"=w361:u8, "Started"=w356:bool)  [unwired: 7 in, 1 out]
        n235 = Array Subset(array=w362, length (row)=w361) -> (w360:string[][])  [unwired: 3 in]
        n236 = Select(t="Executing" ("Cmd Status"), s=w356, f="" ("Cmd Status")) -> (s? t:f=w357:string)
        n237 = local write "Cmd Status"(w357) -> ()
      }
      event "CheckList": Double Click {
        # "Shift clears all"
        # "Update symbols on the listbox"
        n238 = event-data() -> ("PlatMods.Shift"=w368:bool, "Row"=w370:i32)  [unwired: 1 in]
        n239 = case shown="True" w368 {
          tunnel: w370 -> [w374 _]
          tunnel: 1 -> [w373 _]
          frame False {
            n240 = property on="CheckList" class="LstBox (strict)"() -> ("Item Symbols"=w372:i32[])  [unwired: 2 in, 2 out]
            n241 = Replace Array Subset(array=w372, new element=w373, index=w374) -> (w371:i32[])
            n242 = property on="CheckList" class="LstBox (strict)"("Item Symbols"=w371) -> ()  [unwired: 2 in, 2 out]
          }
          frame True {
            w375 = 0 ("Top Row")
            n243 = property on="CheckList" class="LstBox (strict)"() -> ("Number of Rows"=w377:u32)  [unwired: 2 in, 2 out]
            n244 = Initialize Array(0, w377) -> (w376:i32[])
            n245 = property on="CheckList" class="LstBox (strict)"("Top Row"=w375, "Value"=w375, "Item Symbols"=w376) -> ()  [unwired: 2 in, 2 out]
          }
        }
      }
      event "CheckList": Key Down {
        # "Update symbols on the listbox\nLeft and right keys check and uncheck"
        n246 = event-data() -> ("VKey"=w381:T17)  [unwired: 1 in]
        n247 = case shown="\"Left\", \"Right\"" w381 {
          selector: w381 -> [w386 _]
          tunnel: eventvkey."Left" ("VKey") -> [w384 _]
          frame "Left", "Right" {
            n248 = Equal?(x=w384, y=w386) -> (x = y?=w385:bool)
            n249 = Select(t=0, s=w385, f=1) -> (s? t:f=w387:i32)
            n250 = property on="CheckList" class="LstBox (strict)"() -> ("Item Symbols"=w390:i32[])  [unwired: 2 in, 2 out]
            n251 = Replace Array Subset(array=w390, new element=w387, index="CheckList") -> (w389:i32[])
            n252 = property on="CheckList" class="LstBox (strict)"("Item Symbols"=w389) -> ()  [unwired: 2 in, 2 out]
          }
          frame Default {
          }
        }
      }
      event "Motor.Enable": Value Change {
        # "When the test mode otor enable helper is set, update that\ntree row item's value"
        n253 = event-data() -> ("NewVal"=w396:bool)  [unwired: 1 in]
        n254 = Unbundle("Motor") -> ("Value"=w395:dbl)  [unwired: 1 out]
        n255 = Select(t=w395, s=w396, f=0.0) -> (s? t:f=w393:dbl)
        n256 = call <vilib>:"NT Write Number.vi"("Numeric"=w393, "Name"=w392) -> ()  [unwired: 9 in, 1 out]
      }
      event "Test Slider": Value Change {
        # "When the test mode slider helper is set, update that\ntree row item's value"
        n257 = event-data() -> ("NewVal"=w399:dbl)  [unwired: 1 in]
        n258 = call <vilib>:"NT Write Number.vi"("Numeric"=w399, "Name"=w400) -> ()  [unwired: 9 in, 1 out]
      }
      event "On/Off": Value Change {
        # "When the test mode on/off helper value is set, update that\ntree row item's value"
        n259 = event-data() -> ("NewVal"=w404:bool)  [unwired: 1 in]
        n260 = Boolean To (0,1)(Boolean=w404) -> (0, 1=w403:i16)
        n261 = call <vilib>:"NT Write Number.vi"("Numeric"=w403, "Name"=w402) -> ()  [unwired: 9 in, 1 out]
      }
      event "Rev/Fwd": Value Change {
        # "When the test mode helper value for relays is set, update that\ntree row item's value"
        n262 = event-data() -> ("NewVal.Forward"=w412:bool, "NewVal.Reverse"=w411:bool)  [unwired: 1 in]
        n263 = Boolean To (0,1)(Boolean=w412) -> (0, 1=w408:i16)
        n264 = Boolean To (0,1)(Boolean=w411) -> (0, 1=w410:i16)
        n265 = Negate(x=w410) -> (-x=w409:i16)
        n266 = Add(x=w408, y=w409) -> (x+y=w407:i16)
        n267 = call <vilib>:"NT Write Number.vi"("Numeric"=w407, "Name"=w406) -> ()  [unwired: 9 in, 1 out]
      }
      event "Test Ring": Value Change {
        # "When a test mode helper value is selected from the ring,\nset the tree item's variable to the string value"
        n268 = event-data() -> ("NewVal"=w416:u16)  [unwired: 1 in]
        n269 = property on="Test Ring" class="Ring (strict)"() -> ("Strings []"=w417:string[])  [unwired: 2 in, 2 out]
        n270 = Index Array(array=w417, index=w416) -> (element=w415:string)
        n271 = call <vilib>:"NT Write String.vi"("String"=w415, "Name"=w414) -> ()  [unwired: 9 in, 1 out]
      }
      event "Rec Mode": Value Change {
        # "Update globals for recording mode and path to read log from.\nClear when logging and let NetworkTables set path for vision to\nuse."
        n272 = event-data() -> ("NewVal"=w428:enum32{"Stop", "Record", "Playback"})  [unwired: 1 in]
        n273 = global write "WPI_DashboardLogging Global.vi" "Logging Filename"(path "") -> ()
        n274 = global write "WPI_DashboardLogging Global.vi" "Recording"(w428) -> ()
        n275 = case shown="\"Playback\"" w428 {
          tunnel: w427 -> [_ w430 w439]
          tunnel: [_ _ w438] -> w425
          tunnel: [_ _ w437] -> _
          tunnel: w423 -> [_ _ w435]
          tunnel: cluster{i32, i32} {-250, 170} -> [_ _ w434]
          tunnel: [_ _ T18 {"Image Size"=TRUE, "Image Type"=TRUE, "Pixel Value"=TRUE, "ROI Information"=TRUE, "Zoom Factor"=FALSE} ("Image Information Shown:All Elements")] -> w418
          tunnel: [_ _ TRUE ("Zoom Factor")] -> w419
          tunnel: w421 -> [_ _ w431]
          frame Default {
          }
          frame "Stop", "Record" {
            # "Place Window too"
            n276 = invoke class="VI" method="FP.Close"(reference=w430) -> (reference out=w429:refnum<vi>)  [unwired: 2 in, 2 out]
            n277 = invoke class="VI" method="Abort VI"(reference=w429) -> ()  [unwired: 2 in, 3 out]
          }
          frame "Playback" {
            n278 = call "Open Playback Panel.vi"("Offset"=w434, "DB VI Ref"=w435, "Playback in"=w439) -> ("Playback out"=w436:refnum<vi>)  [unwired: 8 in]
            n279 = register-events(w436, w431) -> (reference out=w438:refnum<event-registration>, error out=w437:errorcluster)  [unwired: 2 in]
          }
        }
        n280 = property on="Camera Image Right" class="ImageControl"("Image Information Shown"=w418, "Image Information Visible"=w419) -> ()  [unwired: 2 in, 2 out]
        n281 = property on="Camera Image" class="ImageControl"("Image Information Shown"=w418, "Image Information Visible"=w419) -> ()  [unwired: 2 in, 2 out]
        n282 = call <vilib>:"WPI_DashboardNT Log FieldName Cache.vi"("Operation"=enum16{"Lookup/Add", "Index", "Clear"}."Clear") -> ()  [unwired: 8 in, 3 out]
      }
      event Panel Close {
        w441 = enum32{"Stop", "Record", "Playback"}."Stop" ("Rec Mode")
        # "Playback window has been closed, abort"
        n283 = event-data() -> ()  [unwired: 1 in, 4 out]
        n284 = local write "Rec Mode"(w441) -> ()
        n285 = global write "WPI_DashboardLogging Global.vi" "Recording"(w441) -> ()
      }
      event Panel Close {
        # "Abort playback window and ourself"
        n286 = event-data() -> ()  [unwired: 1 in, 4 out]
        n287 = invoke class="VI" method="FP.Close"(reference=w445) -> (reference out=w444:refnum<vi>)  [unwired: 2 in, 2 out]
        n288 = invoke class="VI" method="Abort VI"(reference=w444) -> (error out=w443:errorcluster)  [unwired: 2 in, 2 out]
        n289 = invoke class="VI" method="Abort VI"(error in=w443) -> ()  [unwired: 2 in, 3 out]
      }
      event User Event {
        n290 = event-data() -> ("IDs"=w452:cluster{"RPC field ID":u16, "Unique ID":u16}, "String"=w451:string)  [unwired: 1 in]
        n291 = Bundle("IDs"=w452, "String"=w451) -> (w450:T9)  [unwired: 1 in]
        n292 = call <vilib>:"Retrieve RPC Response.vi"("RPC Response"=w450) -> ("Output"=w448:string[][])  [unwired: 10 in]
        n293 = Build Array (concatenate)(w446, w448) -> (w447:string[][])
        n294 = local write "Command Params"(w447) -> ()
        n295 = local write "Cmd Status"("" ("Cmd Status")) -> ()
      }
      event "Tree": Double Click {
        n296 = event-data() -> ("PlatMods"=w458:T21, "Tag"=w455:string)  [unwired: 1 in]
        n297 = Unbundle(w458) -> ("Shift"=w457:bool)  [unwired: 4 out]
        n298 = String Subset(string=w455, length (rest)=1 ("length (rest)")) -> (substring=w454:string)  [unwired: 1 in]
        n299 = Not(x=w457) -> (.not. x?=w456:bool)
        n300 = case shown="\"/\"" w454 {
          tunnel: w455 -> [_ w461]
          tunnel: w456 -> [_ w460]
          frame Default {
          }
          frame "/" {
            n301 = call <vilib>:"NT Update Persistence.vi"("Persistence"=w460, "Name"=w461) -> ()  [unwired: 9 in, 1 out]
          }
        }
      }
    }
  }
  n302 = while {
    tunnel: w64 -> [w463]
    i -> [w466]
    stop <- FALSE stop-if-true
    n303 = Wait (ms)(milliseconds to wait=u32 100) -> ()  [unwired: 1 out]
    n304 = case shown="\"Playback\"" "Rec Mode" {
      tunnel: w466 -> [_ _ w481]
      tunnel: [u32 2829099 ("Base Color") u32 11141120 ("Target Color") w470] -> w462
      frame "Stop", Default {
        # "Reset the color, extra updates don't cost much"
      }
      frame "Record" {
      }
      frame "Playback" {
        # "Playback"
        n305 = Quotient & Remainder(x=w481, y=u32 50 ("milliseconds to wait")) -> (x-y*floor(x/y)=w477:u32)  [unwired: 1 out]
        n306 = Divide(x=w477, y=u32 50 ("milliseconds to wait")) -> (x/y=w474:dbl)
        n307 = Multiply(x=6.283185307179586, y=w474) -> (x*y=w479:dbl)
        n308 = Sine(x=w479) -> (sin(x)=w478:dbl)
        n309 = Absolute Value(x=w478) -> (abs(x)=w471:dbl)
        n310 = call "Interpolate RGB Color.vi"("Proportion"=w471, "Target Color"=u32 30976, "Base Color"=u32 2829099) -> ("Result Color"=w470:u32)  [unwired: 8 in]
      }
    }
    n311 = property class="Pane"(reference=w463, "PaneColor"=w462) -> ()  [unwired: 1 in, 2 out]
  }
  n312 = local write "Dashboard Tab"(T2."Drive" ("Dashboard Tab")) -> ()
  n313 = property on="On/Off" class="Bool (strict)"("Visible"=w35) -> ()  [unwired: 2 in, 2 out]
  n314 = property on="Motor" class="Clust (strict)"("Visible"=w35) -> ()  [unwired: 2 in, 2 out]
  n315 = property on="Progress" class="Clust (strict)"("Visible"=w35) -> ()  [unwired: 2 in, 2 out]
  n316 = property on="Test Ring" class="Ring (strict)"("Visible"=w35) -> ()  [unwired: 2 in, 2 out]
  n317 = property on="Rev/Fwd" class="Clust (strict)"("Visible"=w35) -> ()  [unwired: 2 in, 2 out]
  n318 = while {
    tunnel: u16 1741 ("timeout ms (25000)") -> [w483]
    stop <- FALSE stop-if-true
    n319 = TCP Create Listener(10:w483) -> (0:w482:errorcluster, 3:w484:refnum<k5>)  [unwired: 4 in, 1 out]
    n320 = case shown="No Error" w482 {
      selector: w482 -> [w486 _]
      tunnel: w484 -> [w487 _]
      frame No Error {
        n321 = while {
          tunnel: w487 -> [w490]
          tunnel: w486 -> [w489]
          stop <- FALSE stop-if-true
          n322 = TCP Wait On Listener(8:w489, 11:w490) -> (0:w491:errorcluster, 4:w492:refnum<k5>)  [unwired: 2 in, 3 out]
          n323 = local write "TCP"(w492) -> ()
          n324 = case shown="No Error" w491 {
            frame No Error {
            }
            frame Error {
              n325 = Wait (ms)(milliseconds to wait=u32 1000) -> ()  [unwired: 1 out]
            }
          }
        }
      }
      frame Error {
        n326 = Wait (ms)(milliseconds to wait=u32 1000) -> ()  [unwired: 1 out]
      }
    }
  }
  n327 = local write "Command Selection"(u16 0 ("milliseconds to wait")) -> ()
  n328 = local write "Command Params"(string[][] [] ("Command Params")) -> ()
  n329 = global write "WPI_DashboardLogging Global.vi" "Recording"(w58) -> ()
  n330 = local write "Rec Mode"(w58) -> ()
  n331 = while {
    stop <- FALSE stop-if-true
    w495 = "RLL"
    n332 = Equal?(x=WPI_DriverStationAllianceInfo."Blue" ("y"), y=WPI_DriverStationAllianceInfo."Blue") -> (x = y?=w505:bool)
    n333 = String Subset(string=w495, offset (0)=2, length (rest)=1 ("length (rest)")) -> (substring=w517:string)
    n334 = String Subset(string=w495, offset (0)=1, length (rest)=1 ("length (rest)")) -> (substring=w516:string)
    n335 = String Subset(string=w495, offset (0)=0, length (rest)=1 ("length (rest)")) -> (substring=w515:string)
    n336 = Build Array(w517, w516, w515) -> (w514:string[])
    n337 = Equal?(x=w514, y="R") -> (x = y?=w509:bool[])
    n338 = Index Array(array=w509, index=2) -> (element=w503:bool)
    n339 = Index Array(array=w509, index=1) -> (element=w502:bool)
    n340 = Index Array(array=w509, index=0) -> (element=w500:bool)
    n341 = case shown="False" w505 {
      tunnel: w503 -> [w525 w529]
      tunnel: [w525 w528] -> w497
      tunnel: w502 -> [w527 w531]
      tunnel: [w527 w530] -> w501
      tunnel: w500 -> [w526 w533]
      tunnel: [w526 w532] -> w498
      frame False {
      }
      frame True {
        n342 = Not(x=w533) -> (.not. x?=w532:bool)
        n343 = Not(x=w531) -> (.not. x?=w530:bool)
        n344 = Not(x=w529) -> (.not. x?=w528:bool)
      }
    }
    "Opponent Left Switch" <- w498
    "Center Left Scale" <- w501
    "Our Left Team Switch" <- w497
    n345 = Not(x=w497) -> (.not. x?=→"Our Right Team Switch":bool)
    n346 = Not(x=w501) -> (.not. x?=→"Center Right Scale":bool)
    n347 = Not(x=w498) -> (.not. x?=→"Opponent Right Switch":bool)
    n348 = Wait (ms)(milliseconds to wait=u32 20) -> ()  [unwired: 1 out]
  }
  n349 = call <vilib>:"NT Write String.vi"("Name"="Auto Selector") -> ()  [unwired: 10 in, 1 out]
